vi "html_creator_final.vi"() -> ()   [LabVIEW 2014]
panel:
  out "Tab Control":enum32{"title", "body ", "link", "write"}(tab)=enum."write"
  in  "include title":bool
  in  "title":string
  in  "header 2":string
  in  "header 1":string
  in  "italix text":string
  in  "bold letters":string
  in  "plain text":string
  in  "select chiose":T1(ring)
  in  "okey":bool
  in  "include another element":bool
  in  "link it":bool
  in  "name":string
  in  "href":string
  in  "need_atribute":bool
  in  "select atribute (normally href)":bool
  in  "link ok":bool
  in  "folder name":string
  out "status":string
  out "html txet":string
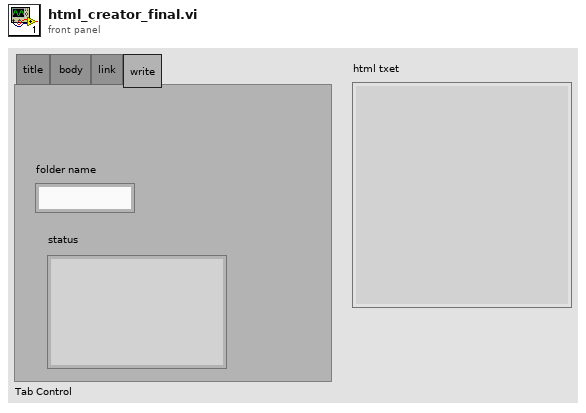
[diagram p1: front panel]
types:
  T1 = enum16{"plain text", "bold", "italic", "header 1", "header 2"}
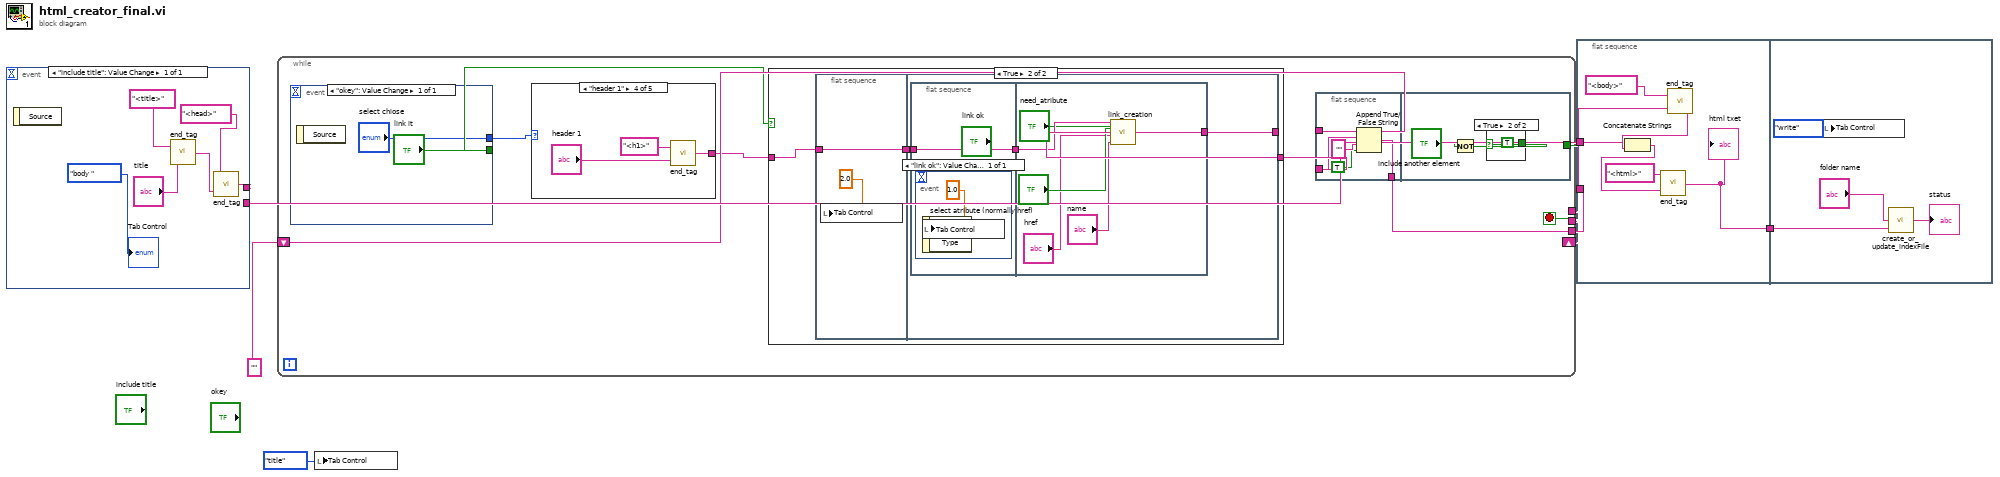
[diagram p0: block diagram]
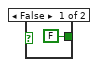
[diagram p2: hidden frame]
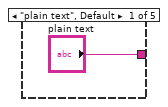
[diagram p3: hidden frame]
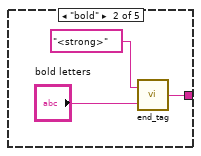
[diagram p4: hidden frame]
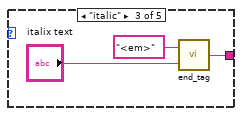
[diagram p5: hidden frame]
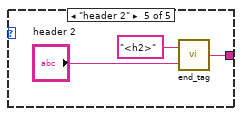
[diagram p6: hidden frame]
diagram:
  n1 = event shown="[0] \"include title\": Value Change" {
    selector: _ -> [_]
    dyn-events: _ -> [_]
    timeout: _ -> [_]
    tunnel: [w7] -> _
    tunnel: [w7] -> w5
    event "include title": Value Change {
      n2 = event-data() -> ()  [unwired: 1 in, 1 out]
      n3 = call "end_tag.vi"("content"="title", "tag"="<title>" ("string")) -> ("full command"=w9:string)
      n4 = call "end_tag.vi"("content"=w9, "tag"="<head>") -> ("full command"=w7:string)
      "Tab Control" <- enum32{"title", "body ", "link", "write"}."body " ("Tab Control")
    }
  }
  n5 = while {
    shift-right: [w15] -> _
    shift-left: "" ("output string") -> [w18]
    tunnel: [w15] -> _
    tunnel: [w15] -> _
    tunnel: [w15] -> w4
    stop <- w14 stop-if-true
    n6 = event shown="[0] \"okey\": Value Change" {
      selector: _ -> [_]
      dyn-events: _ -> [_]
      timeout: _ -> [_]
      tunnel: ["select chiose"] -> w13
      tunnel: ["link it"] -> w12
      event "okey": Value Change {
        n7 = event-data() -> ()  [unwired: 1 in, 1 out]
      }
    }
    n8 = case shown="\"header 1\"" w13 {
      tunnel: ["plain text" w32 w35 w38 w41] -> w17
      frame "plain text", Default {
      }
      frame "bold" {
        n9 = call "end_tag.vi"("content"="bold letters", "tag"="<strong>") -> ("full command"=w32:string)
      }
      frame "italic" {
        n10 = call "end_tag.vi"("content"="italix text", "tag"="<em>") -> ("full command"=w35:string)
      }
      frame "header 1" {
        n11 = call "end_tag.vi"("content"="header 1", "tag"="<h1>") -> ("full command"=w38:string)
      }
      frame "header 2" {
        n12 = call "end_tag.vi"("content"="header 2", "tag"="<h2>") -> ("full command"=w41:string)
      }
    }
    n13 = case shown="True" w12 {
      tunnel: w17 -> [w44 w47]
      tunnel: [w44 w46] -> w16
      frame False {
      }
      frame True {
        n14 = flat-sequence {
          tunnel: w47 -> [w49]
          tunnel: [w49] -> w45
          tunnel: w45 -> [w52]
          tunnel: [w51] -> w46
          frame #0 {
            n15 = local write "Tab Control"(2.0) -> ()
          }
          frame #1 {
            n16 = flat-sequence {
              tunnel: w52 -> [w53]
              tunnel: [w53] -> w50
              tunnel: [w55] -> w51
              tunnel: w50 -> [w60]
              frame #0 {
                n17 = event shown="[0] \"link ok\": Value Change" {
                  selector: _ -> [_]
                  dyn-events: _ -> [_]
                  timeout: _ -> [_]
                  event "link ok": Value Change {
                    n18 = event-data() -> ()  [unwired: 1 in, 2 out]
                    n19 = local write "Tab Control"(1.0) -> ()
                  }
                }
              }
              frame #1 {
                n20 = call "link_creation.vi"("content"=w60, "select atribute"="select atribute (normally href)", "href"="href", "name"="name", "need_atribute"="need_atribute") -> ("result"=w55:string)
              }
            }
          }
        }
      }
    }
    n21 = flat-sequence {
      tunnel: w18 -> [w25]
      tunnel: w16 -> [w23]
      tunnel: [w21] -> w15
      tunnel: [w26] -> w14
      frame #0 {
        n22 = Append True/False String(1:TRUE ("selector"), 2:"", 3:w23, 4:w25) -> (0:w21:string)
      }
      frame #1 {
        n23 = Not(x="include another element") -> (.not. x?=w28:bool)
        n24 = case shown="True" w28 {
          tunnel: [FALSE TRUE] -> w26
          frame False {
          }
          frame True {
          }
        }
      }
    }
  }
  n25 = local write "Tab Control"(enum32{"title", "body ", "link", "write"}."title" ("Tab Control")) -> ()
  n26 = flat-sequence {
    tunnel: w5 -> [w63]
    tunnel: w4 -> [w62]
    tunnel: [w61] -> w2
    tunnel: w2 -> [w71]
    frame #0 {
      n27 = call "end_tag.vi"("content"=w62, "tag"="<body>" ("string")) -> ("full command"=w64:string)
      n28 = Concatenate Strings(w63, w64) -> (w67:string)
      n29 = call "end_tag.vi"("content"=w67, "tag"="<html>") -> ("full command"=w61:string)
      "html txet" <- w61
    }
    frame #1 {
      n30 = local write "Tab Control"(enum32{"title", "body ", "link", "write"}."write" ("Tab Control")) -> ()
      n31 = call "create_or_update_indexFile.vi"("html code"=w71, "folder name"="folder name") -> ("status"=→"status":string)  [unwired: 1 in]
    }
  }
